vi "myRIO_BRIG_RT__timeFPGA.vi"() -> ()   [LabVIEW 2014]
uses:
  <vilib>/Platform/TimedLoop/XDataNode/timing_clust.ctl
  <vilib>/Platform/TimedLoop/XDataNode/nitl_modes.ctl
  <vilib>/Platform/TimedLoop/XDataNode/wakeup.ctl
  <vilib>/myRIO/Common/Instrument Driver Framework/myRIO v1.0/UART/vis/myRIO v1.0 Close UART.vi
  <vilib>/FPGAPlugInAG/myRIO-1900/niLvFpga_Open_myRIO-1900.vi
  <vilib>/rvi/interface/common/dynamic/niFpgaDynamicAddResources.vi
  <vilib>/Utility/error.llb/Error Cluster From Error Code.vi
  <vilib>/rvi/errors/niLvFpgaAdjustHostInterfaceError.vi
  <vilib>/FPGAPlugInAG/Dynamic/niLvFpga_Close_Dynamic.vi
  <vilib>/myRIO/Common/Instrument Driver Framework/Utilities/vis/FPGA Ref Manager.vi
  <vilib>/myRIO/Common/Instrument Driver Framework/myRIO v1.0/myRIO v1.0 Reset FPGA.vi
  <vilib>/myRIO/Common/Instrument Driver Framework/myRIO v1.0/IRQ/vis/myRIO v1.0 IRQ Info FGV.vi
  <vilib>/myRIO/Common/Instrument Driver Framework/myRIO v1.0/IRQ/vis/myRIO v1.0 Timer IRQ Info FGV.vi
  <vilib>/myRIO/Common/Instrument Driver Framework/myRIO v1.0/IRQ/vis/myRIO v1.0 ISR Agent.vi
  <vilib>/rvi/interface/nirviOpenFPGA/nirviOpenFPGA.xnode
  myRIO_BRig_FPGA_v3,51__build.lvbitx
  myRIO_BRig_FPGA_v3,51.vi
  <vilib>/platform/TimedLoop/XDataNode/XDataNode.xnode
  <vilib>/rvi/interface/nirviReadWriteControl/nirviReadWriteControl.xnode
  <vilib>/rvi/interface/nirviCloseFPGA/nirviCloseFPGA.xnode
  <vilib>/myRIO/Instrument Drivers/Utilities/Utilities.lvlib
  NiFpgaLv.dll
  <vilib>/rvi/interface/Simulation/niFpgaSimulationCallBeginRW.vi
  <vilib>/Platform/TimedLoop/XDataNode/XDNodeRunTimeDep.lvlib
panel:
  out "k1__count/ms":dbl
  out "count_timeTrial":u32
  in  "time__ms":i64
  in  "timeTrial":bool
  in  "stop":bool
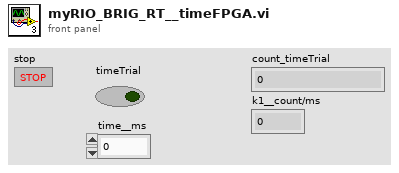
[diagram p1: front panel]
types:
  T1 = typedef "XDNodeRunTimeDep.lvlib/timing_clust.ctl" = cluster{"Expected End [f-1]":u64, "Actual End [f-1]":u64, "Finished Late? [f-1]":bool, "Expected End [i-1]":u64, "Actual End [i-1]":u64, "Finished Late? [i-1]":bool, "Expected Start [i]":u64, "Actual Start [i]":u64, "Expected Start [f]":u64, "Actual Start [f]":u64, "Source Name":string, "Structure Name":string, "Period":i64, "Deadline":i64, "Offset":i64, "Start":i64, "Priority":i32, "Timeout":i32, "Mode":T2, "Wakeup Reason":T3, "Error":errorcluster, "Source Type":string, "Secondary Source Type":string, "Global End Time":u64, "Global Start Time":u64, "Frame Duration":u64, "Iteration Duration":u64, "Assigned CPU":i32, "I/O Scan Engine Mode":u32}
  T2 = typedef "XDNodeRunTimeDep.lvlib/nitl_modes.ctl" = enum32{"No Change", "Process missed periods, maintain original phase", "Discard missed periods, maintain original phase", "Process missed periods, ignore original phase", "Discard missed periods, ignore original phase"}
  T3 = typedef "XDNodeRunTimeDep.lvlib/wakeup.ctl" = enum32{"Normal", "Aborted", "Asynchronous wakeup", "Timing source error", "Timed loop error", "Timeout"}
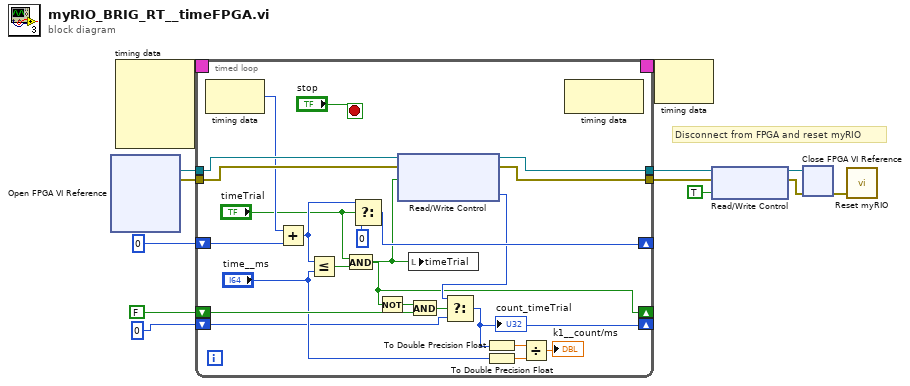
[diagram p0: block diagram]
diagram:
  # "Disconnect from FPGA and reset myRIO"
  n1 = xnode "Open FPGA VI Reference"() -> ("FPGA VI Reference Out"=w9:refnum<k20>, "error out"=w7:errorcluster)  [unwired: 2 in]
  n2 = node-c288() -> (w5:T1)  [unwired: 4 in]
  n3 = timed-loop {
    tunnel: w9 -> [w34]
    tunnel: [w32] -> w8
    tunnel: w7 -> [w33]
    tunnel: [w31] -> w6
    timing: w5 -> [_]
    timing-out: [_] -> w4
    shift-right: [w28] -> _
    shift-left: i64 0 -> [w35]
    shift-right: [w20] -> _
    shift-left: FALSE -> [w24]
    shift-right: [w14] -> _
    shift-left: u32 0 -> [w15]
    stop <- "stop" stop-if-true
    n4 = node-c288() -> (w30:i64)  [unwired: 1 in]
    n5 = Add(x=w30, y=w35) -> (x+y=w29:i64)
    n6 = Less Or Equal?(x=w29, y="time__ms") -> (x <= y?=w26:bool)
    n7 = And(x="timeTrial", y=w26) -> (x .and. y?=w20:bool)
    n8 = Select(t=w29, s="timeTrial", f=i64 0) -> (s? t:f=w28:i64)
    n9 = Not(x=w20) -> (.not. x?=w25:bool)
    n10 = xnode "Read/Write Control"("FPGA VI Reference In"=w34, "error in"=w33, "timeTrial"=w20) -> ("FPGA VI Reference Out"=w32:refnum<k20>, "error out"=w31:errorcluster, "count_timeTrial"=w22:u32)
    n11 = local write "timeTrial"(w20) -> ()
    n12 = And(x=w25, y=w24) -> (x .and. y?=w23:bool)
    n13 = Select(t=w22, s=w23, f=w15) -> (s? t:f=w14:u32)
    "count_timeTrial" <- w14
    n14 = To Double Precision Float(number=w14) -> (double precision float=w19:dbl)
    n15 = To Double Precision Float(number="time__ms") -> (double precision float=w18:dbl)
    n16 = Divide(x=w19, y=w18) -> (x/y=→"k1__count/ms":dbl)
    n17 = node-c288() -> ()  [unwired: 1 in, 1 out]
  }
  n18 = node-c288(w4) -> ()  [unwired: 1 out]
  n19 = xnode "Read/Write Control"("FPGA VI Reference In"=w8, "error in"=w6, "FPGA_Stop"=TRUE) -> ("FPGA VI Reference Out"=w11:refnum<k20>, "error out"=w12:errorcluster)
  n20 = xnode "Close FPGA VI Reference"("FPGA VI Reference In"=w11, "error in"=w12) -> ("error out"=w10:errorcluster)
  n21 = call <vilib>:"Reset myRIO.vi"("error in (no error)"=w10) -> ()  [unwired: 10 in, 1 out]
